vi "rtlsdr_write_config_data.vi"(8 "error in (no error)":errorcluster, 9 "input data":i32, 10 "parameter select":u8, 11 "ref in":refnum<k5>) -> (0 "error out":errorcluster, 3 "ref out":refnum<k5>)   [LabVIEW 2011]
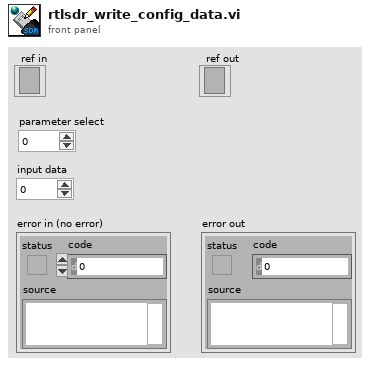
[diagram p1: front panel]
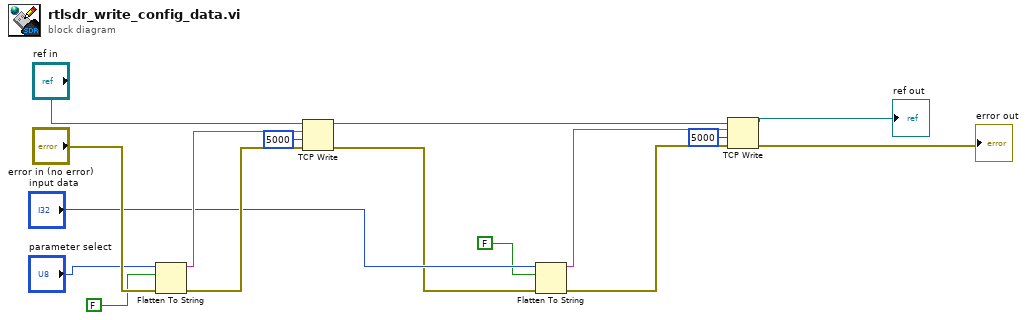
[diagram p0: block diagram]
diagram:
  n1 = Flatten To String(anything="parameter select", prepend array or string size? (T)=FALSE, error in (no error)="error in (no error)") -> (data string=w8:string, error out=w9:errorcluster)  [unwired: 1 in, 1 out]
  n2 = TCP Write(connection ID="ref in", data in=w8, error in (no error)=w9, 9:5000 ("timeout ms (25000)")) -> (connection ID out=w13:refnum<k5>, error out=w5:errorcluster)  [unwired: 1 out]
  n3 = Flatten To String(anything="input data", prepend array or string size? (T)=FALSE, error in (no error)=w5) -> (data string=w3:string, error out=w4:errorcluster)  [unwired: 1 in, 1 out]
  n4 = TCP Write(connection ID=w13, data in=w3, error in (no error)=w4, 9:5000 ("timeout ms (25000)")) -> (connection ID out=→"ref out":refnum<k5>, error out=→"error out":errorcluster)  [unwired: 1 out]
